vi "MGCC_comm_main.vi"() -> ()   [LabVIEW 2016]
doc: "-----------------------------------------------------------------------------------------------------------------------\nCopyright <2019> <The University of Tennessee at Knoxville and the University of Tennessee Research Foundation>\nThis software is released under BSD-3 \nhttps://opensource.org/licenses/BSD-3-Clause \nAdditional license options available at https://utrf.tennessee.edu/industry/sample-agreements/\n-----------------------------------------------------------------------------------------------------------------------"
uses:
  <vilib>/DNP3/DNP3_Master/Operation Mode.ctl
  <vilib>/DNP3/DNP3_Master/Poll Binary Input Variation.ctl
  <vilib>/DNP3/DNP3_Master/Analog Variation.ctl
  <vilib>/DNP3/DNP3_Master/Poll Analog Input Variation.ctl
  <vilib>/DNP3/DNP3_Master/Response Type.ctl
  <vilib>/DNP3/DNP3_Master/Analog Info.ctl
  Global communication output.vi
  Global communication.vi
  MGCC_Global_communication_inputsettings .vi
  <vilib>/Utility/error.llb/Error Cluster From Error Code.vi
  <vilib>/ErrorRing/Error Ring.xnode
  DNP3 communication files/Master Communication Files/DNP3_Master_Station_MGCC.lvlib
  <vilib>/DNP3/DNP3_Master.lvlib
panel:
  out "error out 3":errorcluster
  out "error out 2":errorcluster
  out "error out":errorcluster
  out "Analog Input 2":dbl[](array[numeric])
  out "Analog Input":dbl[](array[numeric])
  in  "LC1_MS_Network_Settings 2":T1={"Outstation IP"="48.26.87.214", "DNP3 Port"=18000, "DNP3 Master Address"=12340, "DNP3 Outstation Address"=54320}
  in  "LC1_MS_DNP3_Settings 2":T6={"Binary Out Mode"=6, "Binary In Variation"=0, "Analog Out Variation"=4, "Analog Out Mode"=6, "Analog In Variation"=6} {"Analog In Variation" items=["Default", "32-bit with Flag", "16-bit with Flag", "32-bit without Flag", "16-bit without Flag", "Single-prec with Flag", "Double-prec with Flag"]; "Analog Out Mode" items=["SBO"=0, "Select"=3, "Operate"=4, "Direct"=5, "Direct No Ack"=6]; "Analog Out Variation" items=["32-bit"=1, "16-bit"=2, "Single-prec"=3, "Double-prec"=4]; "Binary In Variation" items=["Default", "Packed Format", "With Flags"]; "Binary Out Mode" items=["SBO"=0, "Select"=3, "Operate"=4, "Direct"=5, "Direct No Ack"=6]}
  in  "ENABLE MS 2":bool=TRUE
  out "MS SETTINGS CHANGED 2":bool
  out "LC1_MS_TX_Status_Binary 2":T7=enum."Cancel"
  out "LC1_MS_TX_Status_Analog 2":T7=enum."Success"
  out "LC1_MS_RX_Status_Binary 2":T7=enum."Cancel"
  out "LC1_MS_RX_Status_Analog 2":T7=enum."Success"
  out "RESET MS IND 2":bool
  out "Numeric 2":i32=1993
  in  "Poll Enable 2":T8={"En_Rx_An"=TRUE, "En_Tx_An"=TRUE, "En_Rx_Di"=FALSE, "En_Tx_Di"=FALSE}
  in  "RESET MS 2":bool caption="Reset Outstation"
  in  "Poll Enable":T8={"En_Rx_An"=TRUE, "En_Tx_An"=TRUE, "En_Rx_Di"=FALSE, "En_Tx_Di"=FALSE}
  out "Numeric":i32=1993
  out "RESET MS IND":bool
  out "LC1_MS_RX_Status_Analog":T7=enum."Success"
  out "LC1_MS_RX_Status_Binary":T7=enum."Cancel"
  out "LC1_MS_TX_Status_Analog":T7=enum."Success"
  out "LC1_MS_TX_Status_Binary":T7=enum."Cancel"
  out "MS SETTINGS CHANGED":bool
  in  "RESET MS":bool caption="Reset Outstation"
  in  "ENABLE MS":bool=TRUE
  in  "LC1_MS_DNP3_Settings":T6={"Binary Out Mode"=6, "Binary In Variation"=0, "Analog Out Variation"=4, "Analog Out Mode"=6, "Analog In Variation"=6} {"Analog In Variation" items=["Default", "32-bit with Flag", "16-bit with Flag", "32-bit without Flag", "16-bit without Flag", "Single-prec with Flag", "Double-prec with Flag"]; "Analog Out Mode" items=["SBO"=0, "Select"=3, "Operate"=4, "Direct"=5, "Direct No Ack"=6]; "Analog Out Variation" items=["32-bit"=1, "16-bit"=2, "Single-prec"=3, "Double-prec"=4]; "Binary In Variation" items=["Default", "Packed Format", "With Flags"]; "Binary Out Mode" items=["SBO"=0, "Select"=3, "Operate"=4, "Direct"=5, "Direct No Ack"=6]}
  in  "LC1_MS_Network_Settings":T1={"Outstation IP"="48.26.87.213", "DNP3 Port"=18000, "DNP3 Master Address"=12345, "DNP3 Outstation Address"=54321}
  in  "Manually control Relays":bool
  in  "PV on off":bool
  in  "Manually control PV":bool
  in  "BESS on off":bool
  in  "Manually control BESS":bool
  in  "PV Control 2":dbl[](array[numeric])
  in  "BESS Control 2":dbl[](array[numeric])
  out "PV_to_MGCC":dbl[](array[numeric])=[1.0, 0.0, 0.0, 0.005523681640625, 53.744964599609375, 1.0]
  out "BESS_to_MGCC":dbl[](array[numeric])
  out "PV Control":dbl[](array[numeric])=[0.0, 0.0, 0.0, 0.0, 1.0]
  out "BESS Control":dbl[](array[numeric])
  out "Analog output":bool[](array[boolean])
  out "Relay_to_MGCC":dbl[](array[numeric])=[1.0, 0.0006846495220577967, 0.0006873814944592526, 60.0, 60.0, 2.4415619373321533, 6.278271946284167e-10, 6.171677299817231e-08, 0.0, 0.0, 1.0, 0.0005072107423956597, 0.000571776596915075, 60.0, 60.0, 1.551474690437317, -1.6475990891830573e-09, 4.052850770239141e-08, 0.0, 0.0, 0.0, 0.0007539754602994896, 0.0006920237685894376, 60.0, 60.0, 16.837549209594727, -1.7539573670825937e-08, 1.7431260531850167e-09, 0.0, 0.0, 1.0, 0.0006942332269034213, 0.0005977328098535922, 60.0, 60.0, -0.5399612188339233, 1.0809289806270621e-07, 4.634268023936224e-08, 0.0, 0.0, 1.0, 0.0006742547696346213, 0.0008461762451143002, 60.0, 60.0, -2.2255873680114746, 7.23401219348732e-09, 4.018172149719001e-09, 0.0, 0.0, 1.0, 0.0006499041425643916, 0.0007326745193802405, 60.0, 60.0, 46.130165100097656, 3.89349634644345e-08, -5.5225729131179004e-08, 0.0, 0.0, 1.0, 0.0008116208516168967, 0.000729818466957756, 60.0, 60.0, 10.438469886779785, 5.115129284633849e-08, -5.98912622303587e-08, 0.0, 0.0, 1.0, 0.0008432924102113323, 0.0008951967658118954, 60.0, 60.0, 1.8573966026306152, 3.4099801554762813e-09, 4.323229956935685e-08, 0.0, 0.0]
  in  "Relay":bool[](array[boolean])
  # "Settings Changed; Reset to Update"
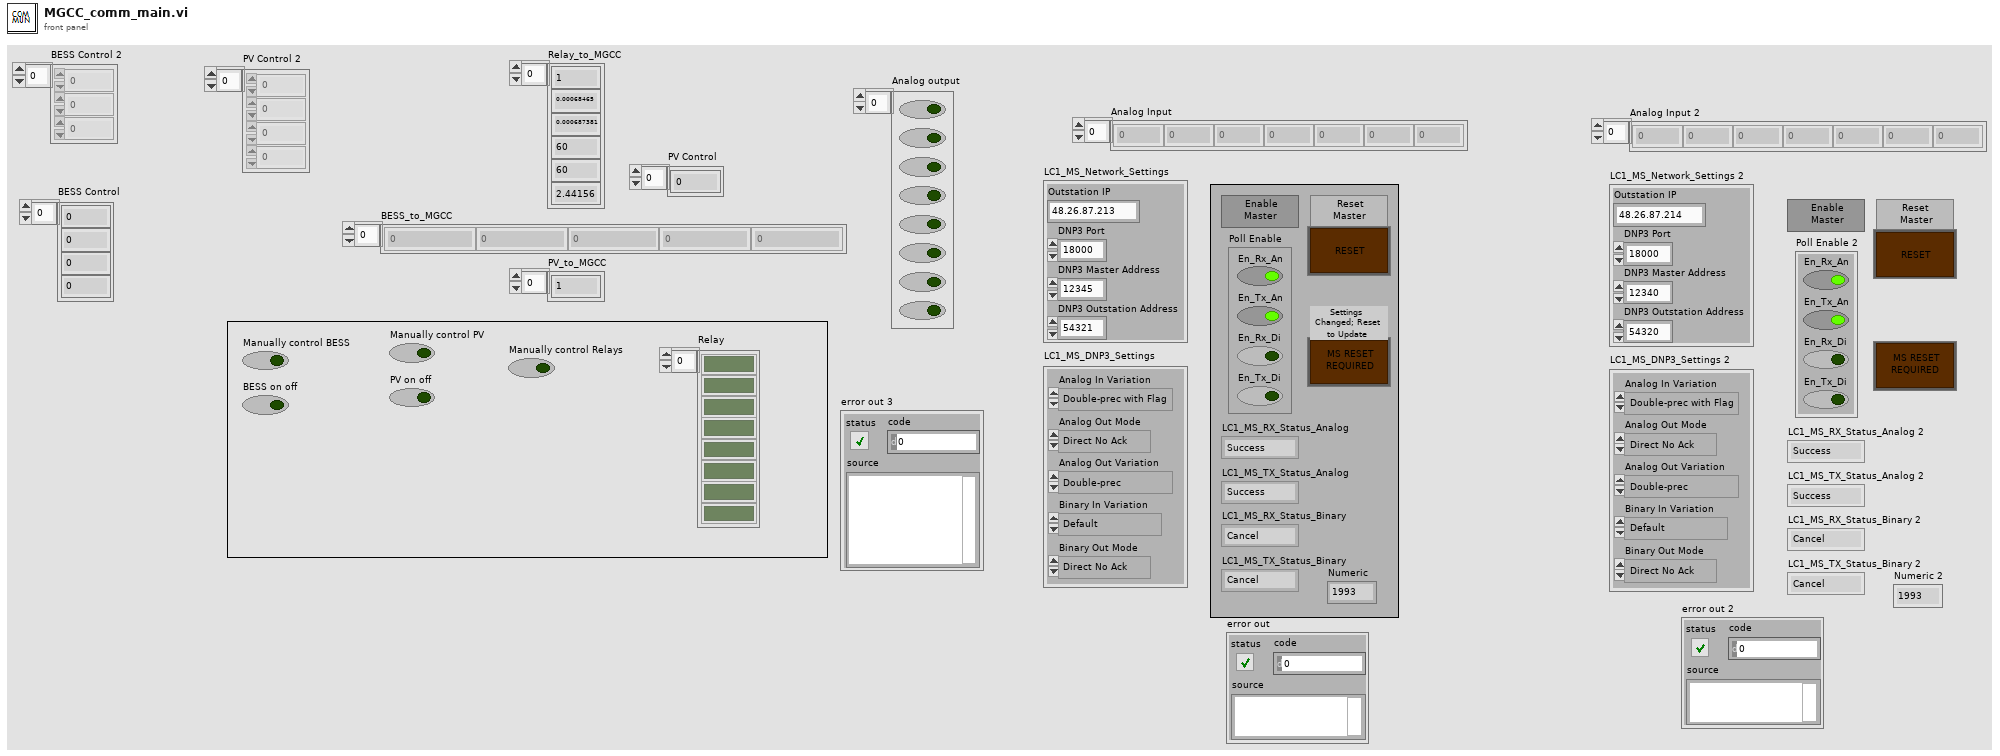
[diagram p1: front panel]
types:
  T1 = cluster{"Outstation IP":string, "DNP3 Port":u16, "DNP3 Master Address":u16, "DNP3 Outstation Address":u16}
  T2 = typedef "DNP3_Master.lvlib/Operation Mode.ctl" = u8
  T3 = typedef "DNP3_Master.lvlib/Poll Binary Input Variation.ctl" = u8
  T4 = typedef "DNP3_Master.lvlib/Analog Variation.ctl" = u8
  T5 = typedef "DNP3_Master.lvlib/Poll Analog Input Variation.ctl" = u8
  T6 = cluster{"Binary Out Mode":T2, "Binary In Variation":T3, "Analog Out Variation":T4, "Analog Out Mode":T2, "Analog In Variation":T5}
  T7 = typedef "DNP3_Master.lvlib/Response Type.ctl" = enum16{"Idle", "Buffering", "Pending", "Success", "Failure", "Mismatch", "Status Code", "IIN", "Timeout", "Cancel"}
  T8 = cluster{"En_Rx_An":bool, "En_Tx_An":bool, "En_Rx_Di":bool, "En_Tx_Di":bool}
  T9 = typedef "DNP3_Master.lvlib/Analog Info.ctl" = cluster{"index":u16, "value":dbl}
  T10 = cluster{"DNP3 channel":refnum<k21>, "DNP3 master":refnum<k21>, "DNP3 master session":refnum<k21>, "DNP3 command":refnum<k21>, "error out":errorcluster}
  T11 = cluster{"response status":T7, "response status":T7, "response status":T7, "response status":T7}
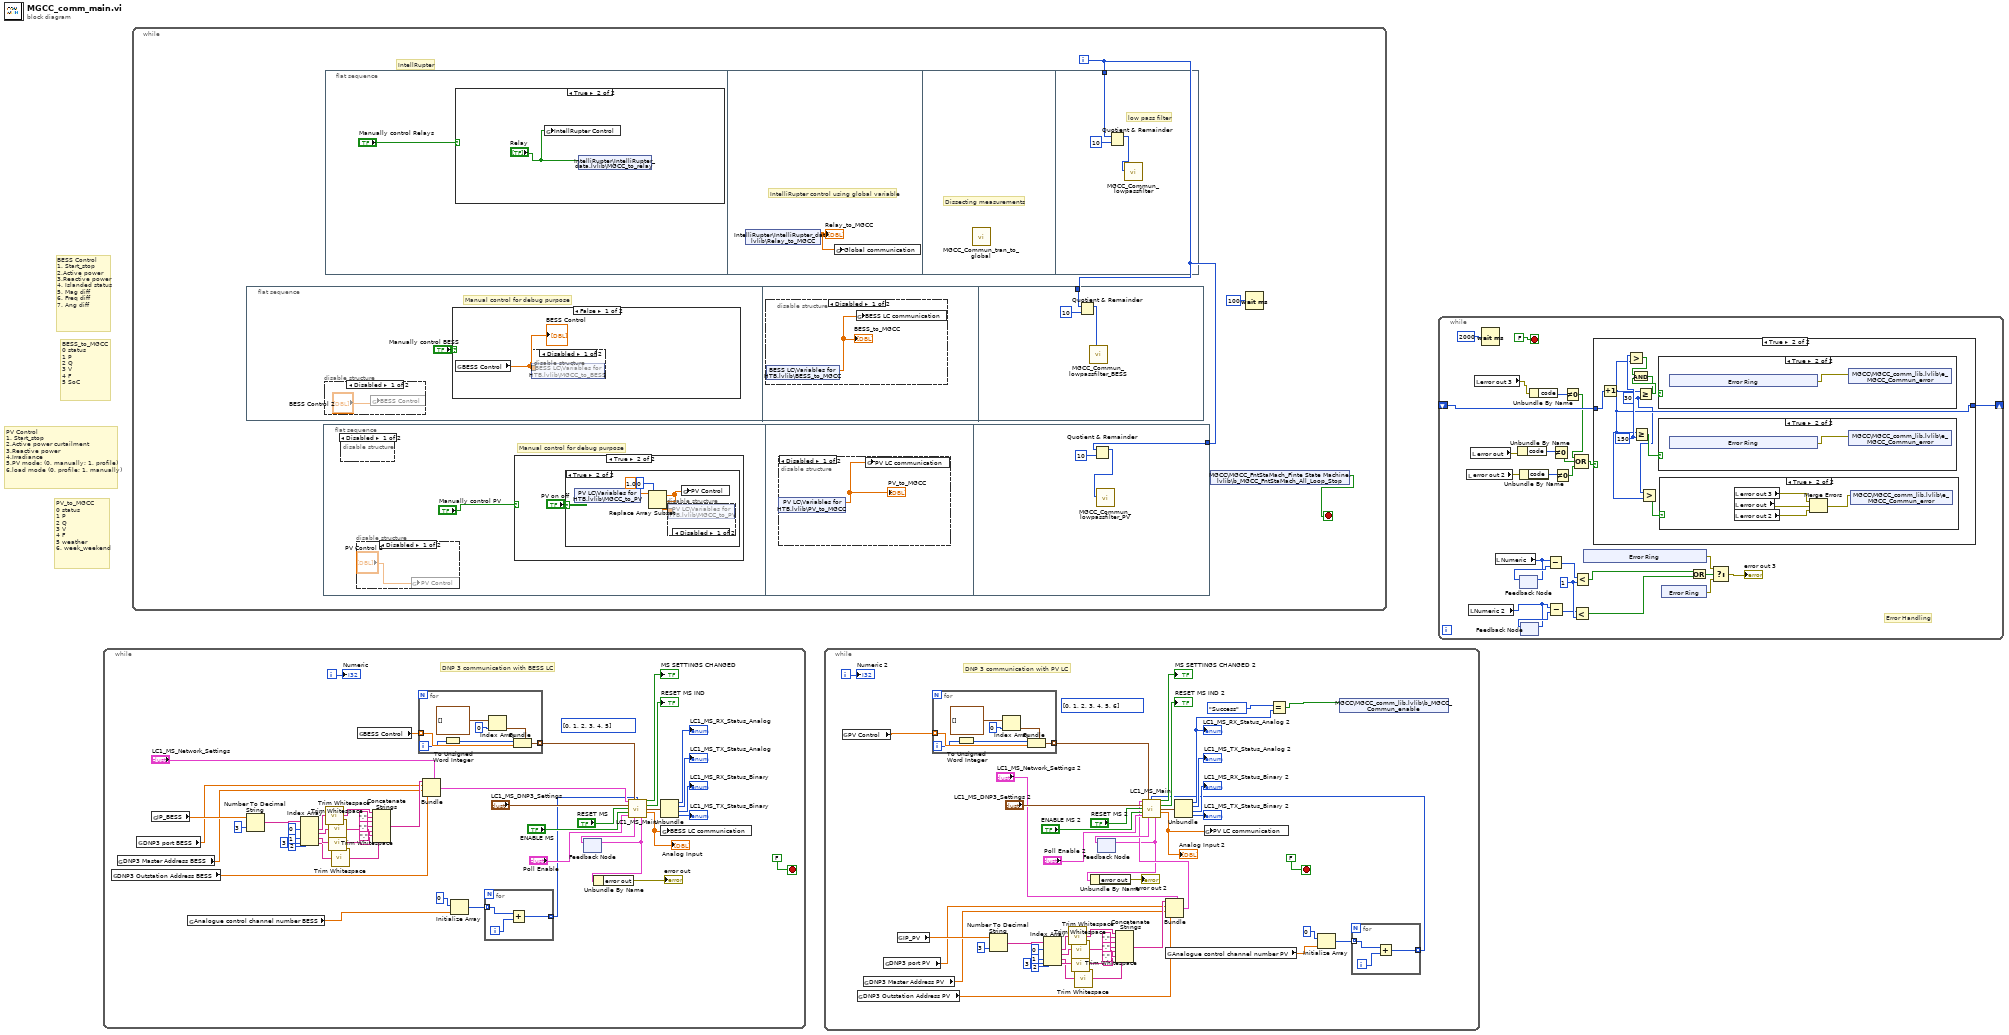
[diagram p0: block diagram]
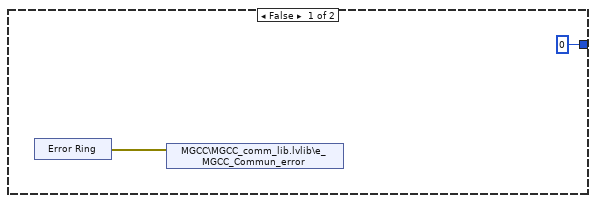
[diagram p2: hidden frame]
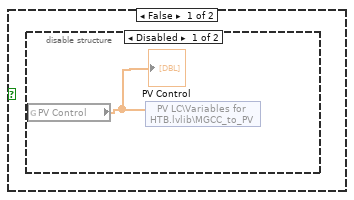
[diagram p6: hidden frame]
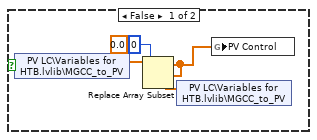
[diagram p8: hidden frame]
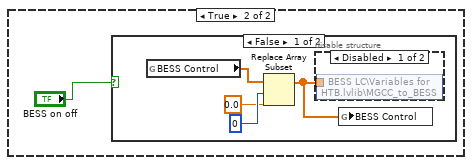
[diagram p14: hidden frame]
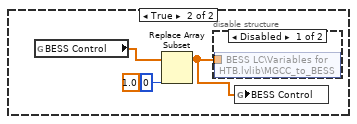
[diagram p16: hidden frame]
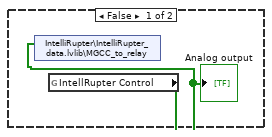
[diagram p20: hidden frame]
diagram:
  # "PV_to_MGCC\n0 status\n1 P\n2 Q\n3 V\n4 F\n5 weather\n6. week_weekend"
  # "BESS_to_MGCC\n0 status\n1 P\n2 Q\n3 V\n4 F\n5 SoC"
  # "PV Control\n1. Start_stop\n2.Active power curtailment\n3.Reactive power\n4.Irradiance\n5.PV mode: (0, manually; 1, profile)\n6.load mode (0, profile; 1, manually)"
  # "BESS Control\n1. Start_stop\n2.Active power\n3.Reactive power\n4. Islanded status\n5. Mag diff\n6. Freq diff\n7. Ang diff"
  n1 = while {
    i -> [w46]
    stop <- FALSE stop-if-true
    (unwired) u16[] [0, 1, 2, 3, 4, 5] ("Analog Input Indexes")
    # "DNP 3 communication with BESS LC"
    n2 = global read "MGCC_Global_communication_inputsettings .vi" "DNP3 Outstation Address BESS"() -> (w7:dbl)
    n3 = global read "MGCC_Global_communication_inputsettings .vi" "DNP3 Master Address BESS"() -> (w8:dbl)
    n4 = global read "MGCC_Global_communication_inputsettings .vi" "DNP3 port BESS"() -> (w9:dbl)
    n5 = global read "MGCC_Global_communication_inputsettings .vi" "IP_BESS"() -> (w11:dbl[])
    n6 = global read "MGCC_Global_communication_inputsettings .vi" "Analogue control channel number BESS"() -> (w3:dbl)
    n7 = Number To Decimal String(number=w11, width (-)=i16 3) -> (decimal integer string=w28:string[])
    n8 = Index Array(array=w28, index #1=0 ("index"), index #2=1 ("index"), index #3=2 ("index"), index #4=3 ("index")) -> (element #1=w20:string, element #2=w18:string, element #3=w16:string, element #4=w14:string)
    n9 = call <vilib>:"Trim Whitespace.vi"("string"=w20) -> ("trimmed string"=w19:string)  [unwired: 1 in]
    n10 = call <vilib>:"Trim Whitespace.vi"("string"=w18) -> ("trimmed string"=w17:string)  [unwired: 1 in]
    n11 = call <vilib>:"Trim Whitespace.vi"("string"=w16) -> ("trimmed string"=w15:string)  [unwired: 1 in]
    n12 = call <vilib>:"Trim Whitespace.vi"("string"=w14) -> ("trimmed string"=w13:string)  [unwired: 1 in]
    n13 = global read "Global communication output.vi" "BESS Control"() -> (w32:dbl[])
    n14 = Concatenate Strings(w19, "." ("string"), w17, "." ("string"), w15, "." ("string"), w13) -> (w10:string)
    n15 = for {
      tunnel: [w57] -> w31 mode=indexing
      tunnel: w32 -> [w52] mode=indexing
      i -> [w51]
      n16 = To Unsigned Word Integer(number=w51) -> (unsigned 16bit integer=w53:u16)
      n17 = Index Array(array=T9[] [] ("values"), index=0) -> (element=w54:T9)
      n18 = Bundle(cluster=w54, "index"=w53, "value"=w52) -> (w57:T9)
    }
    n19 = Bundle(cluster="LC1_MS_Network_Settings", "Outstation IP"=w10, "DNP3 Port"=w9, "DNP3 Master Address"=w8, "DNP3 Outstation Address"=w7) -> (w29:T1)
    n20 = Initialize Array(0, w3) -> (w5:i32[])
    n21 = for {
      tunnel: w5 -> [w50] mode=indexing
      tunnel: [w48] -> w4 mode=indexing
      i -> [w49]
      n22 = Add(x=w50, y=w49) -> (x+y=w48:i32)
    }
    n23 = feedback #1() -> (w41:T10)  [unwired: 1 in]
    n24 = call "LC1_MS_Main.vi"("MS_Network_Settings"=w29, "Analog Output"=w31, "Analog Input Indexes"=w4, "input cluster"="LC1_MS_DNP3_Settings", "MS_RESET"="RESET MS", "MS_ENABLE"="ENABLE MS", "Poll Enable"="Poll Enable", "DNP3 Session feedback"=w41) -> ("MS_SETTINGS_CHANGED"=→"MS SETTINGS CHANGED":bool, "MS_RESET_IND"=→"RESET MS IND":bool, "Cluster"=w34:T11, "Analog Input"=w33:dbl[], "DNP3 Session"=w2:T10)  [unwired: 2 in, 1 out]
    "Analog Input" <- w33
    n25 = feedback-in #1(w2) -> ()
    n26 = Unbundle By Name(w2) -> ("error out"=→"error out":errorcluster)
    n27 = Unbundle(w34) -> ("response status"=→"LC1_MS_RX_Status_Analog":T7, "response status"=→"LC1_MS_TX_Status_Analog":T7, "response status"=→"LC1_MS_RX_Status_Binary":T7, "response status"=→"LC1_MS_TX_Status_Binary":T7)
    n28 = global write "Global communication.vi" "BESS LC communication"(w33) -> ()
    "Numeric" <- w46
  }
  n29 = while {
    i -> [w59]
    stop <- w60 stop-if-true
    # "IntellRupter"
    n30 = flat-sequence {
      tunnel: w59 -> [w95]
      frame #0 {
        # "Manual control for debug purpose"
        n31 = disable-structure shown="Disabled" {
          frame Disabled {
            n32 = global write "Global communication output.vi" "BESS Control"("BESS Control 2") -> ()
          }
          frame Enabled {
          }
        }
        n33 = case shown="False" "Manually control BESS" {
          frame False {
            n34 = global read "Global communication output.vi" "BESS Control"() -> (w79:dbl[])
            "BESS Control" <- w79
            n35 = disable-structure shown="Disabled" {
              disable-tunnel: w79 -> [w80 _]
              frame Disabled {
                n36 = shared-variable "BESS LC\\Variables for HTB.lvlib\\MGCC_to_BESS"(w80) -> ()  [unwired: 1 in, 1 out]
              }
              frame Enabled {
              }
            }
          }
          frame True {
            n37 = case shown="False" "BESS on off" {
              frame False {
                n38 = global read "Global communication output.vi" "BESS Control"() -> (w82:dbl[])
                n39 = Replace Array Subset(array=w82, new element=0.0 ("new element/subarray"), index=0) -> (w83:dbl[])
                n40 = disable-structure shown="Disabled" {
                  disable-tunnel: w83 -> [w86 _]
                  frame Disabled {
                    n41 = shared-variable "BESS LC\\Variables for HTB.lvlib\\MGCC_to_BESS"(w86) -> ()  [unwired: 1 in, 1 out]
                  }
                  frame Enabled {
                  }
                }
                n42 = global write "Global communication output.vi" "BESS Control"(w83) -> ()
              }
              frame True {
                n43 = global read "Global communication output.vi" "BESS Control"() -> (w87:dbl[])
                n44 = Replace Array Subset(array=w87, new element=1.0 ("new element/subarray"), index=0) -> (w88:dbl[])
                n45 = disable-structure shown="Disabled" {
                  disable-tunnel: w88 -> [w91 _]
                  frame Disabled {
                    n46 = shared-variable "BESS LC\\Variables for HTB.lvlib\\MGCC_to_BESS"(w91) -> ()  [unwired: 1 in, 1 out]
                  }
                  frame Enabled {
                  }
                }
                n47 = global write "Global communication output.vi" "BESS Control"(w88) -> ()
              }
            }
          }
        }
      }
      frame #1 {
        n48 = disable-structure shown="Disabled" {
          frame Disabled {
            n49 = shared-variable "BESS LC\\Variables for HTB.lvlib\\BESS_to_MGCC"() -> (w93:dbl[])  [unwired: 1 in, 1 out]
            "BESS_to_MGCC" <- w93
            n50 = global write "Global communication.vi" "BESS LC communication"(w93) -> ()
          }
          frame Enabled {
          }
        }
      }
      frame #2 {
        n51 = Quotient & Remainder(x=w95, y=10) -> (x-y*floor(x/y)=w94:i32)  [unwired: 1 out]
        n52 = call "MGCC_Commun_lowpassfilter_BESS.vi"("Col"=w94) -> ()  [unwired: 11 in]
      }
    }
    n53 = flat-sequence {
      tunnel: w59 -> [w76]
      frame #0 {
        # "Manual control for debug purpose"
        n54 = disable-structure shown="Disabled" {
          frame Disabled {
          }
          frame Enabled {
          }
        }
        n55 = disable-structure shown="Disabled" {
          frame Disabled {
            n56 = global write "Global communication output.vi" "PV Control"("PV Control 2") -> ()
          }
          frame Enabled {
          }
        }
        n57 = case shown="True" "Manually control PV" {
          frame False {
            n58 = disable-structure shown="Disabled" {
              frame Disabled {
                n59 = global read "Global communication output.vi" "PV Control"() -> (w62:dbl[])
                "PV Control" <- w62
                n60 = shared-variable "PV LC\\Variables for HTB.lvlib\\MGCC_to_PV"(w62) -> ()  [unwired: 1 in, 1 out]
              }
              frame Enabled {
              }
            }
          }
          frame True {
            n61 = case shown="True" "PV on off" {
              frame False {
                n62 = shared-variable "PV LC\\Variables for HTB.lvlib\\MGCC_to_PV"() -> (w67:dbl[])  [unwired: 1 in, 1 out]
                n63 = Replace Array Subset(array=w67, new element=0.0 ("new element/subarray"), index=0) -> (w64:dbl[])
                n64 = shared-variable "PV LC\\Variables for HTB.lvlib\\MGCC_to_PV"(w64) -> ()  [unwired: 1 in, 1 out]
                n65 = global write "Global communication output.vi" "PV Control"(w64) -> ()
              }
              frame True {
                n66 = shared-variable "PV LC\\Variables for HTB.lvlib\\MGCC_to_PV"() -> (w71:dbl[])  [unwired: 1 in, 1 out]
                n67 = Replace Array Subset(array=w71, new element=1.0 ("new element/subarray"), index=0) -> (w68:dbl[])
                n68 = disable-structure shown="Disabled" {
                  disable-tunnel: w68 -> [w72 _]
                  frame Disabled {
                    n69 = shared-variable "PV LC\\Variables for HTB.lvlib\\MGCC_to_PV"(w72) -> ()  [unwired: 1 in, 1 out]
                  }
                  frame Enabled {
                  }
                }
                n70 = global write "Global communication output.vi" "PV Control"(w68) -> ()
              }
            }
          }
        }
      }
      frame #1 {
        n71 = disable-structure shown="Disabled" {
          frame Disabled {
            n72 = shared-variable "PV LC\\Variables for HTB.lvlib\\PV_to_MGCC"() -> (w74:dbl[])  [unwired: 1 in, 1 out]
            "PV_to_MGCC" <- w74
            n73 = global write "Global communication.vi" "PV LC communication"(w74) -> ()
          }
          frame Enabled {
          }
        }
      }
      frame #2 {
        n74 = Quotient & Remainder(x=w76, y=10) -> (x-y*floor(x/y)=w75:i32)  [unwired: 1 out]
        n75 = call "MGCC_Commun_lowpassfilter_PV.vi"("Col"=w75) -> ()  [unwired: 11 in]
      }
    }
    n76 = flat-sequence {
      tunnel: w59 -> [w103]
      frame #0 {
        n77 = case shown="True" "Manually control Relays" {
          frame False {
            n78 = global read "Global communication output.vi" "IntellRupter Control"() -> (w98:bool[])
            "Analog output" <- w98
            n79 = shared-variable "IntelliRupter\\IntelliRupter_data.lvlib\\MGCC_to_relay"(w98) -> ()  [unwired: 1 in, 1 out]
          }
          frame True {
            n80 = global write "Global communication output.vi" "IntellRupter Control"("Relay") -> ()
            n81 = shared-variable "IntelliRupter\\IntelliRupter_data.lvlib\\MGCC_to_relay"("Relay") -> ()  [unwired: 1 in, 1 out]
          }
        }
      }
      frame #1 {
        # "IntelliRupter control using global variable"
        n82 = shared-variable "IntelliRupter\\IntelliRupter_data.lvlib\\Relay_to_MGCC"() -> (w100:dbl[])  [unwired: 1 in, 1 out]
        "Relay_to_MGCC" <- w100
        n83 = global write "Global communication.vi" "Global communication"(w100) -> ()
      }
      frame #2 {
        # "Dissecting measurements"
        n84 = call "MGCC_Commun_tran_to_global.vi"() -> ()  [unwired: 12 in]
      }
      frame #3 {
        # "low pass filter"
        n85 = Quotient & Remainder(x=w103, y=10) -> (x-y*floor(x/y)=w101:i32)  [unwired: 1 out]
        n86 = call "MGCC_Commun_lowpassfilter.vi"("Col"=w101) -> ()  [unwired: 11 in]
      }
    }
    n87 = shared-variable "MGCC\\MGCC_FntStaMach_Finte State Machine.lvlib\\b_MGCC_FntStaMach_All_Loop_Stop"() -> (w60:bool)  [unwired: 1 in, 1 out]
    n88 = Wait (ms)(milliseconds to wait=u32 100) -> ()  [unwired: 1 out]
  }
  n89 = while {
    i -> [w151]
    stop <- FALSE stop-if-true
    (unwired) u16[] [0, 1, 2, 3, 4, 5, 6] ("Analog Input Indexes")
    # "DNP 3 communication with PV LC"
    n90 = global read "Global communication output.vi" "PV Control"() -> (w138:dbl[])
    n91 = global read "MGCC_Global_communication_inputsettings .vi" "DNP3 Outstation Address PV"() -> (w112:dbl)
    n92 = global read "MGCC_Global_communication_inputsettings .vi" "DNP3 Master Address PV"() -> (w113:dbl)
    n93 = global read "MGCC_Global_communication_inputsettings .vi" "DNP3 port PV"() -> (w114:dbl)
    n94 = global read "MGCC_Global_communication_inputsettings .vi" "IP_PV"() -> (w116:dbl[])
    n95 = for {
      tunnel: [w162] -> w139 mode=indexing
      tunnel: w138 -> [w157] mode=indexing
      i -> [w156]
      n96 = To Unsigned Word Integer(number=w156) -> (unsigned 16bit integer=w158:u16)
      n97 = Index Array(array=T9[] [] ("values"), index=0) -> (element=w159:T9)
      n98 = Bundle(cluster=w159, "index"=w158, "value"=w157) -> (w162:T9)
    }
    n99 = Number To Decimal String(number=w116, width (-)=i16 3) -> (decimal integer string=w133:string[])
    n100 = Index Array(array=w133, index #1=0 ("index"), index #2=1 ("index"), index #3=2 ("index"), index #4=3 ("index")) -> (element #1=w125:string, element #2=w123:string, element #3=w121:string, element #4=w119:string)
    n101 = call <vilib>:"Trim Whitespace.vi"("string"=w125) -> ("trimmed string"=w124:string)  [unwired: 1 in]
    n102 = call <vilib>:"Trim Whitespace.vi"("string"=w123) -> ("trimmed string"=w122:string)  [unwired: 1 in]
    n103 = call <vilib>:"Trim Whitespace.vi"("string"=w121) -> ("trimmed string"=w120:string)  [unwired: 1 in]
    n104 = call <vilib>:"Trim Whitespace.vi"("string"=w119) -> ("trimmed string"=w118:string)  [unwired: 1 in]
    n105 = feedback #2() -> (w146:T10)  [unwired: 1 in]
    n106 = Concatenate Strings(w124, "." ("string"), w122, "." ("string"), w120, "." ("string"), w118) -> (w115:string)
    n107 = Bundle(cluster="LC1_MS_Network_Settings 2", "Outstation IP"=w115, "DNP3 Port"=w114, "DNP3 Master Address"=w113, "DNP3 Outstation Address"=w112) -> (w110:T1)
    n108 = global read "MGCC_Global_communication_inputsettings .vi" "Analogue control channel number PV"() -> (w109:dbl)
    n109 = Initialize Array(0, w109) -> (w107:i32[])
    n110 = for {
      tunnel: w107 -> [w155] mode=indexing
      tunnel: [w153] -> w106 mode=indexing
      i -> [w154]
      n111 = Add(x=w155, y=w154) -> (x+y=w153:i32)
    }
    n112 = call "LC1_MS_Main.vi"("MS_Network_Settings"=w110, "Analog Output"=w139, "Analog Input Indexes"=w106, "input cluster"="LC1_MS_DNP3_Settings 2", "MS_RESET"="RESET MS 2", "MS_ENABLE"="ENABLE MS 2", "Poll Enable"="Poll Enable 2", "DNP3 Session feedback"=w146) -> ("MS_SETTINGS_CHANGED"=→"MS SETTINGS CHANGED 2":bool, "MS_RESET_IND"=→"RESET MS IND 2":bool, "Cluster"=w140:T11, "Analog Input"=w137:dbl[], "DNP3 Session"=w104:T10)  [unwired: 2 in, 1 out]
    "Analog Input 2" <- w137
    n113 = Unbundle By Name(w104) -> ("error out"=→"error out 2":errorcluster)
    n114 = feedback-in #2(w104) -> ()
    n115 = Unbundle(w140) -> ("response status"=w135:T7, "response status"=→"LC1_MS_TX_Status_Analog 2":T7, "response status"=→"LC1_MS_RX_Status_Binary 2":T7, "response status"=→"LC1_MS_TX_Status_Binary 2":T7)
    "LC1_MS_RX_Status_Analog 2" <- w135
    n116 = global write "Global communication.vi" "PV LC communication"(w137) -> ()
    n117 = Equal?(x=Response_Type."Success" ("LC1_MS_RX_Status_Analog 2"), y=w135) -> (x = y?=w134:bool)
    n118 = shared-variable "MGCC\\MGCC_comm_lib.lvlib\\b_MGCC_Commun_enable"(w134) -> ()  [unwired: 1 in, 1 out]
    "Numeric 2" <- w151
  }
  n119 = while {
    shift-right: [w187] -> _
    shift-left: _ -> [w186]
    stop <- FALSE stop-if-true
    w173 = 1 ("y")
    # "Error Handling"
    n120 = local read "error out 2"() -> (w183:errorcluster)
    n121 = local read "Numeric 2"() -> (w169:i32)
    n122 = local read "error out"() -> (w184:errorcluster)
    n123 = local read "error out 3"() -> (w163:errorcluster)
    n124 = Wait (ms)(milliseconds to wait=u32 2000) -> ()  [unwired: 1 out]
    n125 = local read "Numeric"() -> (w167:i32)
    n126 = Unbundle By Name(w184) -> ("code"=w181:i32)
    n127 = Unbundle By Name(w183) -> ("code"=w182:i32)
    n128 = feedback #3() -> (w168:i32)  [unwired: 1 in]
    n129 = feedback-in #3(w167) -> ()
    n130 = feedback #4() -> (w170:i32)  [unwired: 1 in]
    n131 = feedback-in #4(w169) -> ()
    n132 = Unbundle By Name(w163) -> ("code"=w185:i32)
    n133 = Subtract(x=w167, y=w168) -> (x-y=w171:i32)
    n134 = Subtract(x=w169, y=w170) -> (x-y=w172:i32)
    n135 = Not Equal To 0?(x=w181) -> (x != 0?=w179:bool)
    n136 = Not Equal To 0?(x=w182) -> (x != 0?=w178:bool)
    n137 = Not Equal To 0?(x=w185) -> (x != 0?=w180:bool)
    n138 = Less?(x=w172, y=w173) -> (x < y?=w175:bool)
    n139 = Less?(x=w171, y=w173) -> (x < y?=w174:bool)
    n140 = Compound Arithmetic op=OR(w180, w179, w178) -> (w177:bool)
    n141 = xnode "Error Ring"() -> ("error out"=w166:errorcluster)
    n142 = case shown="True" w177 {
      tunnel: [0 w201] -> w187
      tunnel: w186 -> [_ w207]
      frame False {
        n143 = xnode "Error Ring"() -> ("error out"=w196:errorcluster)
        n144 = shared-variable "MGCC\\MGCC_comm_lib.lvlib\\e_MGCC_Commun_error"(w196) -> ()  [unwired: 1 in, 1 out]
      }
      frame True {
        w202 = 150 ("y")
        w200 = 30 ("y")
        n145 = Increment(x=w207) -> (x+1=w201:i32)
        n146 = Greater?(x=w202, y=w201) -> (0:w204:bool)
        n147 = Greater Or Equal?(x=w201, y=w202) -> (x >= y?=w206:bool)
        n148 = Greater Or Equal?(x=w201, y=w200) -> (x >= y?=w205:bool)
        n149 = And(x=w204, y=w205) -> (x .and. y?=w203:bool)
        n150 = Greater?(x=w200, y=w201) -> (0:w199:bool)
        n151 = case shown="True" w203 {
          frame False {
          }
          frame True {
            n152 = xnode "Error Ring"() -> ("error out"=w218:errorcluster)
            n153 = shared-variable "MGCC\\MGCC_comm_lib.lvlib\\e_MGCC_Commun_error"(w218) -> ()  [unwired: 1 in, 1 out]
          }
        }
        n154 = case shown="True" w206 {
          frame False {
          }
          frame True {
            n155 = xnode "Error Ring"() -> ("error out"=w212:errorcluster)
            n156 = shared-variable "MGCC\\MGCC_comm_lib.lvlib\\e_MGCC_Commun_error"(w212) -> ()  [unwired: 1 in, 1 out]
          }
        }
        n157 = case shown="True" w199 {
          frame False {
          }
          frame True {
            n158 = local read "error out 3"() -> (w211:errorcluster)
            n159 = local read "error out"() -> (w210:errorcluster)
            n160 = local read "error out 2"() -> (w209:errorcluster)
            n161 = Merge Errors(w211, w210, w209) -> (w208:errorcluster)
            n162 = shared-variable "MGCC\\MGCC_comm_lib.lvlib\\e_MGCC_Commun_error"(w208) -> ()  [unwired: 1 in, 1 out]
          }
        }
      }
    }
    n163 = xnode "Error Ring"() -> ("error out"=w165:errorcluster)
    n164 = Or(x=w174, y=w175) -> (x .or. y?=w164:bool)
    n165 = Select(t=w166, s=w164, f=w165) -> (s? t:f=→"error out 3":errorcluster)
  }
